vi "Read Sink Settings.vi"(0 "Event Source in":refnum<class "Event Source.lvclass">, 1 "Sink Name":string, 5 "error in (no error)":errorcluster) -> (14 "Event Source out":refnum<class "Event Source.lvclass">, 19 "error out":errorcluster)   [LabVIEW 2016, in "Event Source.lvlib" / "Event Source.lvclass"]
doc: "Allows to set the Sink behaviour by setting the following flags\n\n\"Exclude From Broadcast\"\nmessage originating form another sink will not be broadcasted to the sink being cosidered\n\"Paused\"\nThe sink will not send events and will not receive them anymore\n\"Receive only\"\nThe sing will receive events but not sany any"
uses:
  Event Source.lvclass
  Event Source.lvclass/Event Source.ctl
  Sink Details.ctl
  <vilib>/ActorFramework/Message Enqueuer/Message Enqueuer.lvclass
  Sink Settings.ctl
panel:
  out "Sink Not Found":bool
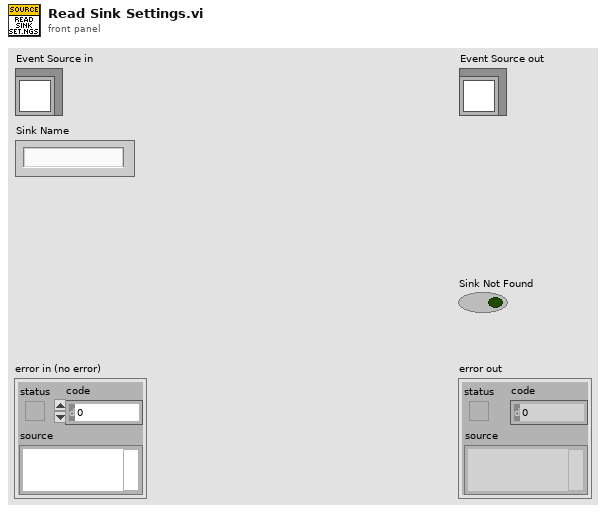
[diagram p1: front panel]
types:
  T1 = typedef "Event Source.lvlib/Event Source.lvclass/Sink Settings Event Ref.ctl" = refnum<user-event>
  T2 = typedef "Event Source.lvlib/Event Source.lvclass/Sink Settings.ctl" = cluster{"Exclude From Broadcast":bool, "Receive Only":bool, "Paused":bool}
  T3 = typedef "Event Source.lvlib/Event Source.lvclass/Sink Details.ctl" = cluster{"Exclude From Broadcast":bool, "Receive Only":bool, "Paused":bool, "Sink Enqueuer":refnum<class "Message Enqueuer.lvclass">}
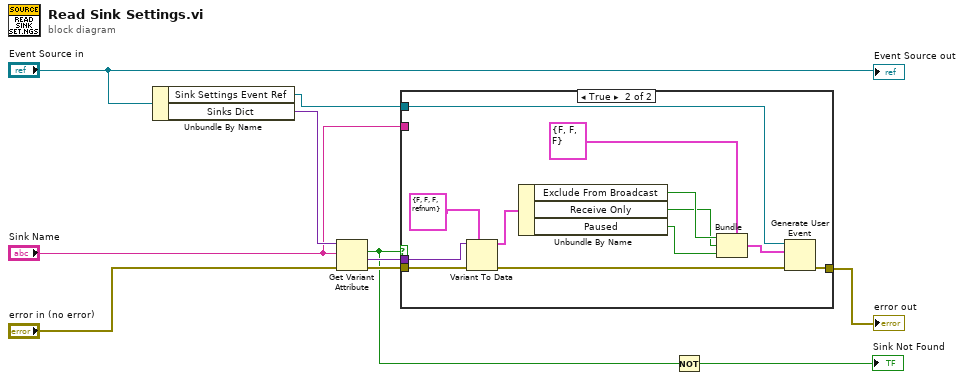
[diagram p0: block diagram]
diagram:
  n1 = Unbundle By Name("Event Source in") -> ("Sink Settings Event Ref"=w1:T1, "Sinks Dict"=w8:variant)
  n2 = Get Variant Attribute(Variant=w8, name="Sink Name", error in="error in (no error)") -> (found=w3:bool, value=w9:variant, error out=w10:errorcluster)  [unwired: 1 in, 1 out]
  n3 = case shown="True" w3 {
    tunnel: w9 -> [_ w22]
    tunnel: w10 -> [w11 w23]
    tunnel: [w11 w14] -> w4
    tunnel: "Sink Name" -> [_ _]
    tunnel: w1 -> [_ w13]
    frame False {
    }
    frame True {
      n4 = Variant To Data(error in=w23, type=T3 {"Exclude From Broadcast"=FALSE, "Receive Only"=FALSE, "Paused"=FALSE, "Sink Enqueuer"=refnum} ("Message Enqueuer"), Variant=w22) -> (data=w20:T3, error out=w15:errorcluster)
      n5 = Unbundle By Name(w20) -> ("Exclude From Broadcast"=w18:bool, "Receive Only"=w17:bool, "Paused"=w16:bool)
      n6 = Bundle(cluster=T2 {"Exclude From Broadcast"=FALSE, "Receive Only"=FALSE, "Paused"=FALSE} ("Sink Settings"), "Exclude From Broadcast"=w18, "Receive Only"=w17, "Paused"=w16) -> (w12:T2)
      n7 = Generate User Event(user event=w13, event data cluster=w12, error in=w15) -> (error out=w14:errorcluster)  [unwired: 1 in, 1 out]
    }
  }
  "error out" <- w4
  n8 = Not(x=w3) -> (.not. x?=→"Sink Not Found":bool)
  "Event Source out" <- "Event Source in"
